vi "String to String Array.vi"(8 "error in (no error)":errorcluster, 11 "String received":string) -> (0 "error out":errorcluster, 3 "Array Data":string[](array[string]))   [LabVIEW 2016, in "Environment Chamber.lvlib" / "Climatic Chamber.lvlib"]
uses:
  Climatic Chamber.lvlib
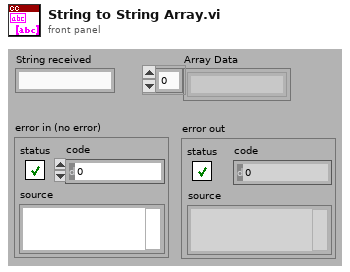
[diagram p1: front panel]
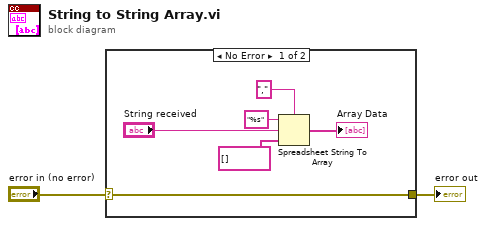
[diagram p0: block diagram]
diagram:
  n1 = case shown="No Error" "error in (no error)" {
    selector: "error in (no error)" -> [w3 w9]
    tunnel: [w3 w9] -> w1
    frame No Error {
      n2 = Spreadsheet String To Array(delimiter (Tab)=",", format string="%s", spreadsheet string="String received", array type (2D Dbl)=string[] []) -> (array=→"Array Data":string[])
    }
    frame Error {
    }
  }
  "error out" <- w1
